vi "Generate waveform.vi"(8 "error in (no error)":errorcluster, 11 "Galvo in":refnum<class "ImagingModeSPIM.lvclass">) -> (0 "error out":errorcluster, 2 "Array":variant[](array[variant]), 3 "Galvo out":refnum<class "ImagingModeSPIM.lvclass">)   [LabVIEW 2012, in "ImagingModeSPIM.lvclass"]
uses:
  ImagingModeSPIM.lvclass
  ImagingModeSPIM.lvclass/ImagingModeSPIM.ctl
  Controls/wavelength_ring.ctl
  <vilib>/measure/NI_MABase.lvlib
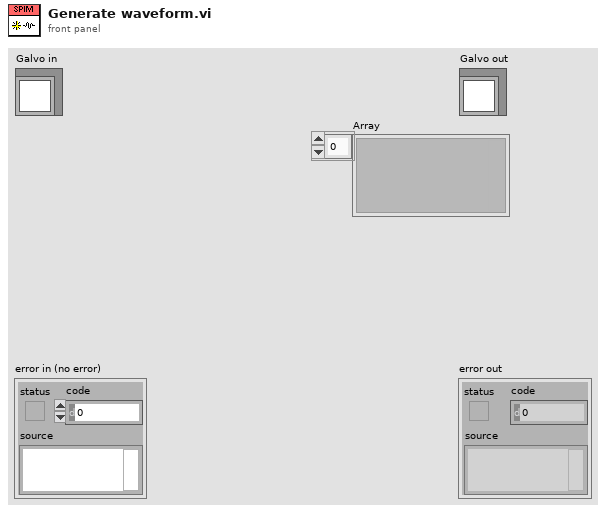
[diagram p1: front panel]
types:
  T1 = typedef "ImagingModeSPIM.lvclass/number of channels.ctl" = enum16{"empty", "double sided + PC", "double sided + WFS"}
  T2 = typedef "ImagingModeSPIM.lvclass/waveform data.ctl" = cluster{"Amplitude":dbl[unit], "Offset":dbl[unit], "Phase":dbl[unit], "Duty cycle":dbl, "sampling info":cluster{"Fs":dbl, "#s":dbl}, "frequency":dbl[unit], "Waveform type":T3}
  T3 = typedef "ImagingModeSPIM.lvclass/waveform_enum.ctl" = enum16{"triangular", "step", "sawtooth", "sinusodial", "skewed sawtooth"}
  T4 = typedef "ImagingModeSPIM.lvclass/Pockels cell.ctl" = cluster{"Wavelength":T5, "digital ratio":dbl, "pulses per pixel":i32, "frequency":dbl[unit], "amplitude":dbl[unit], "phase":dbl[unit], "sampling info":cluster{"Fs":dbl, "#s":dbl}}
  T5 = typedef "ImagingModeSPIM.lvclass/wavelength_ring.ctl" = dbl
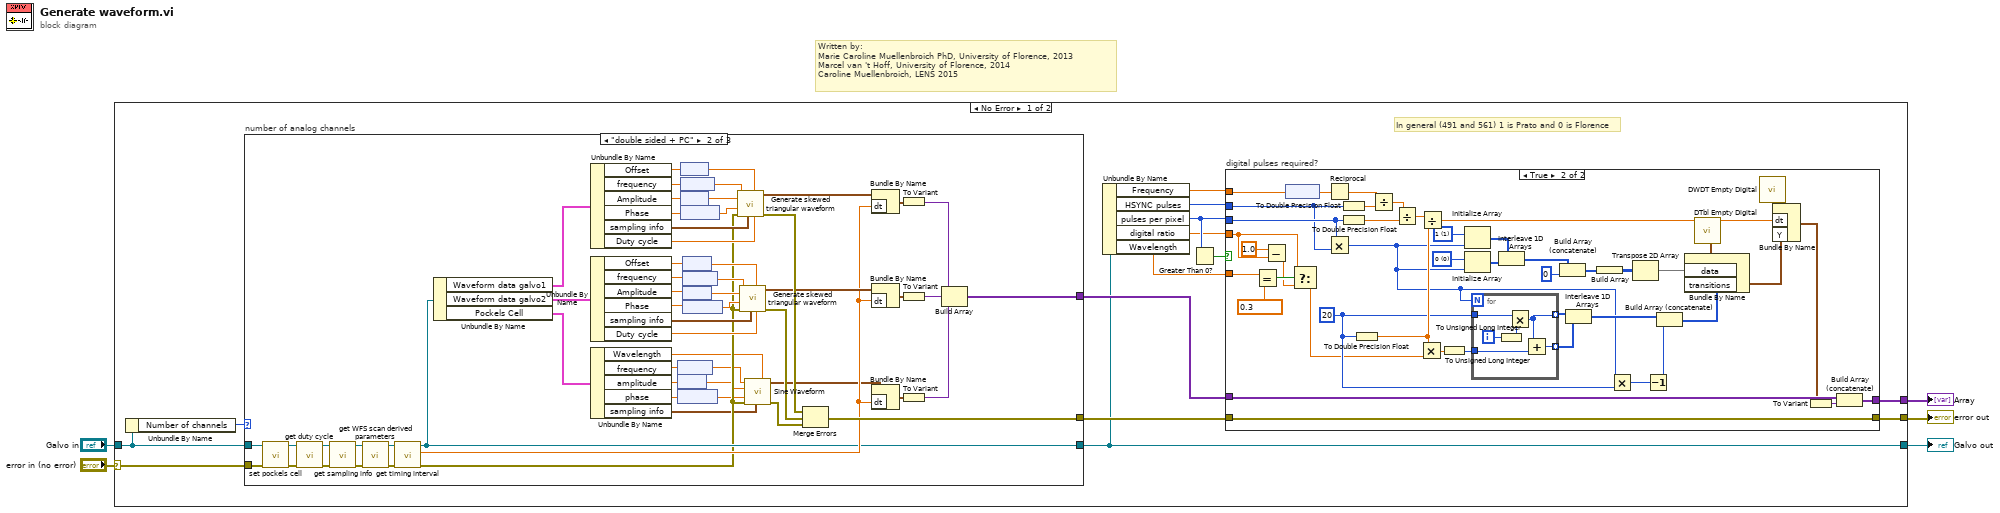
[diagram p0: block diagram]
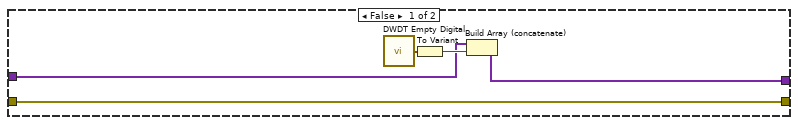
[diagram p2: hidden frame]
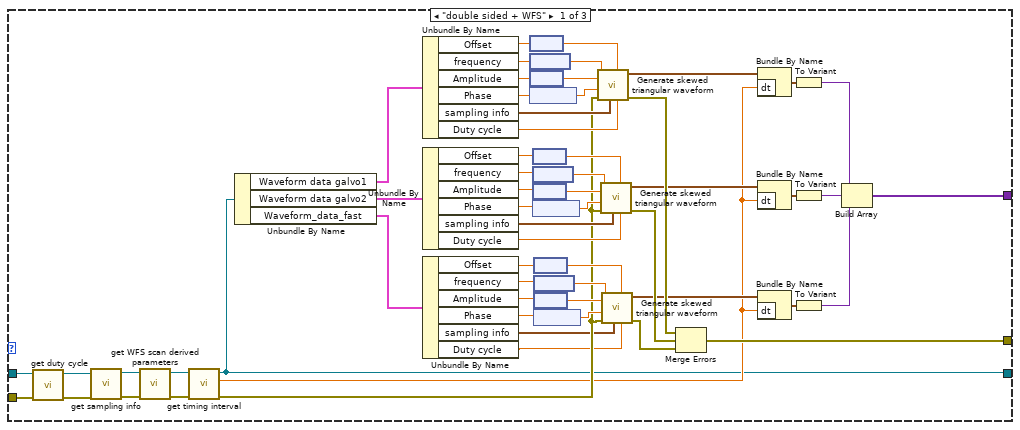
[diagram p3: hidden frame]
diagram:
  # "Written by:\nMarie Caroline Muellenbroich PhD, University of Florence, 2013 \nMarcel van 't Hoff, University of Florence, 2014\nCaroline Muellenbroich, LENS 2015"
  n1 = case shown="No Error" "error in (no error)" {
    selector: "error in (no error)" -> [w19 w195]
    tunnel: [w12 w195] -> w5
    tunnel: [w7 w194] -> w4
    tunnel: "Galvo in" -> [w8 w194]
    tunnel: [w17 _] -> w3
    frame No Error {
      # "In general (491 and 561) 1 is Prato and 0 is Florence"
      n2 = Unbundle By Name(w8) -> ("Number of channels"=w10:T1)
      n3 = case "number of analog channels" shown="\"double sided + PC\"" w10 {
        tunnel: [w133 w191 w193] -> w18
        tunnel: w19 -> [w126 w146 w193]
        tunnel: [w132 w190 _] -> w16
        tunnel: w8 -> [w125 w148 w192]
        tunnel: [w76 w149 w192] -> w7
        frame "double sided + WFS" {
          n4 = call-dynamic "get duty cycle.vi"("error in (no error)"=w126, "ImagingModeSPIM in"=w125) -> ("error out"=w124:errorcluster, "ImagingModeSPIM out"=w123:refnum<class "ImagingModeSPIM.lvclass">)  [unwired: 8 in]
          n5 = call-dynamic "get sampling info.vi"("error in (no error)"=w124, "ImagingModeSPIM in"=w123) -> ("error out"=w122:errorcluster, "ImagingModeSPIM out"=w120:refnum<class "ImagingModeSPIM.lvclass">)  [unwired: 8 in]
          n6 = call-dynamic "get WFS scan derived parameters.vi"("error in (no error)"=w122, "ImagingModeSPIM in"=w120) -> ("error out"=w121:errorcluster, "ImagingModeSPIM out"=w119:refnum<class "ImagingModeSPIM.lvclass">)  [unwired: 8 in]
          n7 = call-dynamic "get timing interval.vi"("error in (no error)"=w121, "ImagingModeSPIM in"=w119) -> ("error out"=w88:errorcluster, "dt"=w77:dbl, "ImagingModeSPIM out"=w76:refnum<class "ImagingModeSPIM.lvclass">)  [unwired: 7 in]
          n8 = Unbundle By Name(w76) -> ("Waveform data galvo1"=w127:T2, "Waveform data galvo2"=w106:T2, "Waveform_data_fast"=w105:T2)
          n9 = Unbundle By Name(w127) -> ("Offset"=w118:dbl[unit], "frequency"=w116:dbl[unit], "Amplitude"=w114:dbl[unit], "Phase"=w112:dbl[unit], "sampling info"=w109:cluster{"Fs":dbl, "#s":dbl}, "Duty cycle"=w108:dbl)
          n10 = Unbundle By Name(w106) -> ("Offset"=w100:dbl[unit], "frequency"=w99:dbl[unit], "Amplitude"=w98:dbl[unit], "Phase"=w97:dbl[unit], "sampling info"=w96:cluster{"Fs":dbl, "#s":dbl}, "Duty cycle"=w95:dbl)
          n11 = Unbundle By Name(w105) -> ("Offset"=w87:dbl[unit], "frequency"=w86:dbl[unit], "Amplitude"=w85:dbl[unit], "Phase"=w84:dbl[unit], "sampling info"=w83:cluster{"Fs":dbl, "#s":dbl}, "Duty cycle"=w82:dbl)
          n12 = node(w118) -> (w117:dbl)
          n13 = node(w116) -> (w115:dbl)
          n14 = node(w114) -> (w113:dbl)
          n15 = node(w112) -> (w111:dbl)
          n16 = node(w100) -> (w101:dbl)
          n17 = node(w99) -> (w102:dbl)
          n18 = node(w98) -> (w103:dbl)
          n19 = node(w97) -> (w104:dbl)
          n20 = node(w87) -> (w92:dbl)
          n21 = node(w86) -> (w91:dbl)
          n22 = node(w85) -> (w90:dbl)
          n23 = node(w84) -> (w89:dbl)
          n24 = call "Generate skewed triangular waveform.vi"("Duty cycle (%)"=w108, "Offset"=w117, "sampling info"=w109, "error in (no error)"=w88, "Phase"=w111, "Amplitude"=w113, "Frequency"=w115) -> ("error out"=w110:errorcluster, "Waveform"=w107:waveform(dbl))  [unwired: 3 in]
          n25 = call "Generate skewed triangular waveform.vi"("Duty cycle (%)"=w95, "Offset"=w101, "sampling info"=w96, "error in (no error)"=w88, "Phase"=w104, "Amplitude"=w103, "Frequency"=w102) -> ("error out"=w94:errorcluster, "Waveform"=w93:waveform(dbl))  [unwired: 3 in]
          n26 = call "Generate skewed triangular waveform.vi"("Duty cycle (%)"=w82, "Offset"=w92, "sampling info"=w83, "error in (no error)"=w88, "Phase"=w89, "Amplitude"=w90, "Frequency"=w91) -> ("error out"=w81:errorcluster, "Waveform"=w80:waveform(dbl))  [unwired: 3 in]
          n27 = Merge Errors(w110, w94, w81) -> (w133:errorcluster)
          n28 = Bundle By Name(cluster=w107, "dt"=w77) -> (w128:waveform(dbl))
          n29 = Bundle By Name(cluster=w93, "dt"=w77) -> (w129:waveform(dbl))
          n30 = Bundle By Name(cluster=w80, "dt"=w77) -> (w78:waveform(dbl))
          n31 = To Variant(anything=w128) -> (Variant=w130:variant)
          n32 = To Variant(anything=w129) -> (Variant=w131:variant)
          n33 = To Variant(anything=w78) -> (Variant=w79:variant)
          n34 = Build Array(w130, w131, w79) -> (w132:variant[])
        }
        frame "double sided + PC" {
          n35 = call-dynamic "set pockels cell.vi"("error in (no error)"=w146, "ImagingModeSPIM in"=w148) -> ("error out"=w145:errorcluster, "ImagingModeSPIM out"=w147:refnum<class "ImagingModeSPIM.lvclass">)  [unwired: 8 in]
          n36 = call-dynamic "get duty cycle.vi"("error in (no error)"=w145, "ImagingModeSPIM in"=w147) -> ("error out"=w184:errorcluster, "ImagingModeSPIM out"=w183:refnum<class "ImagingModeSPIM.lvclass">)  [unwired: 8 in]
          n37 = call-dynamic "get sampling info.vi"("error in (no error)"=w184, "ImagingModeSPIM in"=w183) -> ("error out"=w182:errorcluster, "ImagingModeSPIM out"=w180:refnum<class "ImagingModeSPIM.lvclass">)  [unwired: 8 in]
          n38 = call-dynamic "get WFS scan derived parameters.vi"("error in (no error)"=w182, "ImagingModeSPIM in"=w180) -> ("error out"=w181:errorcluster, "ImagingModeSPIM out"=w179:refnum<class "ImagingModeSPIM.lvclass">)  [unwired: 8 in]
          n39 = call-dynamic "get timing interval.vi"("error in (no error)"=w181, "ImagingModeSPIM in"=w179) -> ("error out"=w144:errorcluster, "dt"=w150:dbl, "ImagingModeSPIM out"=w149:refnum<class "ImagingModeSPIM.lvclass">)  [unwired: 7 in]
          n40 = Unbundle By Name(w149) -> ("Waveform data galvo1"=w185:T2, "Waveform data galvo2"=w166:T2, "Pockels Cell"=w165:T4)
          n41 = Unbundle By Name(w185) -> ("Offset"=w178:dbl[unit], "frequency"=w176:dbl[unit], "Amplitude"=w174:dbl[unit], "Phase"=w172:dbl[unit], "sampling info"=w169:cluster{"Fs":dbl, "#s":dbl}, "Duty cycle"=w168:dbl)
          n42 = Unbundle By Name(w166) -> ("Offset"=w160:dbl[unit], "frequency"=w159:dbl[unit], "Amplitude"=w158:dbl[unit], "Phase"=w157:dbl[unit], "sampling info"=w156:cluster{"Fs":dbl, "#s":dbl}, "Duty cycle"=w155:dbl)
          n43 = Unbundle By Name(w165) -> ("Wavelength"=w142:T5, "frequency"=w141:dbl[unit], "amplitude"=w139:dbl[unit], "phase"=w137:dbl[unit], "sampling info"=w135:cluster{"Fs":dbl, "#s":dbl})
          n44 = node(w141) -> (w140:dbl)
          n45 = node(w139) -> (w138:dbl)
          n46 = node(w137) -> (w136:dbl)
          n47 = node(w178) -> (w177:dbl)
          n48 = node(w176) -> (w175:dbl)
          n49 = node(w174) -> (w173:dbl)
          n50 = node(w172) -> (w171:dbl)
          n51 = node(w160) -> (w161:dbl)
          n52 = node(w159) -> (w162:dbl)
          n53 = node(w158) -> (w163:dbl)
          n54 = node(w157) -> (w164:dbl)
          n55 = call "Generate skewed triangular waveform.vi"("Duty cycle (%)"=w168, "Offset"=w177, "sampling info"=w169, "error in (no error)"=w144, "Phase"=w171, "Amplitude"=w173, "Frequency"=w175) -> ("error out"=w170:errorcluster, "Waveform"=w167:waveform(dbl))  [unwired: 3 in]
          n56 = call "Generate skewed triangular waveform.vi"("Duty cycle (%)"=w155, "Offset"=w161, "sampling info"=w156, "error in (no error)"=w144, "Phase"=w164, "Amplitude"=w163, "Frequency"=w162) -> ("error out"=w154:errorcluster, "Waveform"=w153:waveform(dbl))  [unwired: 3 in]
          n57 = call <vilib>:"Sine Waveform.vi"("offset"=w142, "sampling info"=w135, "error in (no error)"=w144, "phase"=w136, "amplitude"=w138, "frequency"=w140) -> ("error out"=w143:errorcluster, "signal out"=w134:waveform(dbl))  [unwired: 4 in]
          n58 = Merge Errors(w170, w154, w143) -> (w191:errorcluster)
          n59 = Bundle By Name(cluster=w167, "dt"=w150) -> (w186:waveform(dbl))
          n60 = Bundle By Name(cluster=w153, "dt"=w150) -> (w187:waveform(dbl))
          n61 = Bundle By Name(cluster=w134, "dt"=w150) -> (w151:waveform(dbl))
          n62 = To Variant(anything=w186) -> (Variant=w188:variant)
          n63 = To Variant(anything=w187) -> (Variant=w189:variant)
          n64 = To Variant(anything=w151) -> (Variant=w152:variant)
          n65 = Build Array(w188, w189, w152) -> (w190:variant[])
        }
        frame Default {
        }
      }
      n66 = Unbundle By Name(w7) -> ("Frequency"=w15:dbl[unit], "HSYNC pulses"=w14:i32, "pulses per pixel"=w13:i32, "digital ratio"=w11:dbl, "Wavelength"=w6:T5)
      n67 = Greater Than 0?(x=w13) -> (x > 0?=w9:bool)
      n68 = case "digital pulses required?" shown="True" w9 {
        tunnel: w13 -> [_ w35]
        tunnel: [w24 w51] -> w12
        tunnel: w18 -> [w24 w51]
        tunnel: [w20 w64] -> w17
        tunnel: w16 -> [w21 w65]
        tunnel: w15 -> [_ w69]
        tunnel: w14 -> [_ w32]
        tunnel: w11 -> [_ w27]
        tunnel: w6 -> [_ w31]
        frame False {
          n69 = call <vilib>:"DWDT Empty Digital.vi"() -> ("digital waveform out"=w22:digitalwaveform)  [unwired: 5 in]
          n70 = To Variant(anything=w22) -> (Variant=w23:variant)
          n71 = Build Array (concatenate)(w21, w23) -> (w20:variant[])
        }
        frame True {
          w30 = T5 0.3 items=["405nm"=0.24, "445nm"=0.26, "491nm"=0.29, "515nm"=0.3, "561nm"=0.33] ("y")
          w36 = u32 20 ("ratio step size")
          w53 = u8 0 items=["0", "1", "Z", "L", "H", "X", "T", "V"] ("value 2")
          w52 = u8 1 items=["0", "1", "Z", "L", "H", "X", "T", "V"] ("value 2")
          n72 = Equal?(x=w31, y=w30) -> (x = y?=w28:bool)
          n73 = Subtract(x=1.0, y=w27) -> (x-y=w26:dbl)
          n74 = node(w69) -> (w68:dbl)
          n75 = Select(t=w27, s=w28, f=w26) -> (s? t:f=w25:dbl)
          n76 = Reciprocal(x=w68) -> (1/x=w67:dbl)
          n77 = Multiply(x=w35, y=w32) -> (x*y=w33:i32)
          n78 = To Double Precision Float(number=w32) -> (double precision float=w66:dbl)
          n79 = To Double Precision Float(number=w35) -> (double precision float=w62:dbl)
          n80 = To Double Precision Float(number=w36) -> (double precision float=w47:dbl)
          n81 = Divide(x=w67, y=w66) -> (x/y=w63:dbl)
          n82 = Divide(x=w63, y=w62) -> (x/y=w46:dbl)
          n83 = Multiply(x=w47, y=w25) -> (x*y=w57:dbl)
          n84 = Divide(x=w46, y=w47) -> (x/y=w45:dbl)
          n85 = To Unsigned Long Integer(number=w57) -> (unsigned 32bit integer=w60:u32)
          n86 = Initialize Array(w52, w33) -> (w55:u8[])
          n87 = Initialize Array(w53, w33) -> (w56:u8[])
          n88 = for {
            N: w33 -> [_]
            tunnel: w60 -> [w73]
            tunnel: w36 -> [w75]
            tunnel: [w72] -> w58 mode=indexing
            tunnel: [w71] -> w59 mode=indexing
            i -> [w74]
            n89 = To Unsigned Long Integer(number=w74) -> (unsigned 32bit integer=w70:u32)
            n90 = Multiply(x=w75, y=w70) -> (x*y=w72:u32)
            n91 = Add(x=w72, y=w73) -> (x+y=w71:u32)
          }
          n92 = Interleave 1D Arrays(w55, w56) -> (w41:u8[])
          n93 = Build Array (concatenate)(w41, u8 0 ("value 2")) -> (w40:u8[])
          n94 = Interleave 1D Arrays(w58, w59) -> (w39:u32[])
          n95 = Build Array(w40) -> (w54:u8[][])
          n96 = Multiply(x=w33, y=w36) -> (x*y=w37:u32)
          n97 = Transpose 2D Array(2D array=w54) -> (transposed array=w43:u8[][])
          n98 = Decrement(x=w37) -> (x-1=w34:u32)
          n99 = Build Array (concatenate)(w39, w34) -> (w38:u32[])
          n100 = call <vilib>:"DTbl Empty Digital.vi"() -> ("digital data"=w50:digitaldata)  [unwired: 5 in]
          n101 = Bundle By Name(cluster=w50, "data"=w43, "transitions"=w38) -> (w48:digitaldata)
          n102 = call <vilib>:"DWDT Empty Digital.vi"() -> ("digital waveform out"=w49:digitalwaveform)  [unwired: 5 in]
          n103 = Bundle By Name(cluster=w49, "dt"=w45, "Y"=w48) -> (w61:digitalwaveform)
          n104 = To Variant(anything=w61) -> (Variant=w44:variant)
          n105 = Build Array (concatenate)(w65, w44) -> (w64:variant[])
        }
      }
    }
    frame Error {
    }
  }
  "error out" <- w5
  "Galvo out" <- w4
  "Array" <- w3
